vi "Message Logger.vi"() -> ()   [LabVIEW 2011, in "Messenging.lvlib" / "Message Logger.lvclass"]
uses:
  Message Logger.lvclass
  Parallel Process.lvclass
  Interprocess Messenger/Receiver/MGR (Receive type).lvclass
  Interprocess Messenger/TextVarientMessage/MSG.lvclass
  MessageLoggerMessage/MessageLoggerMessage.lvclass
  <vilib>/Utility/miscctls.llb/LVRowAndColumnUnsignedTypeDef.ctl
  Interprocess Messenger/Send/Send.lvclass
panel:
  out "Table":string[][](table)
  in  "Startup Message":refnum<class "MSG.lvclass">
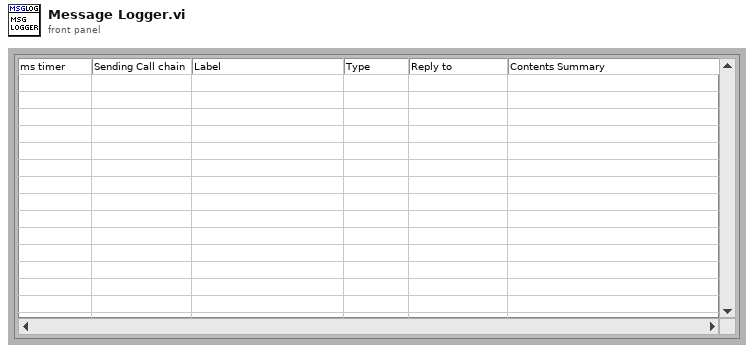
[diagram p1: front panel]
types:
  T1 = typedef "LVRowAndColumnUnsignedTypeDef.ctl" = cluster{"Row":u32, "Column":u32}
  T2 = cluster{"Timeout":i32, "Table":string[][], "index":i32}
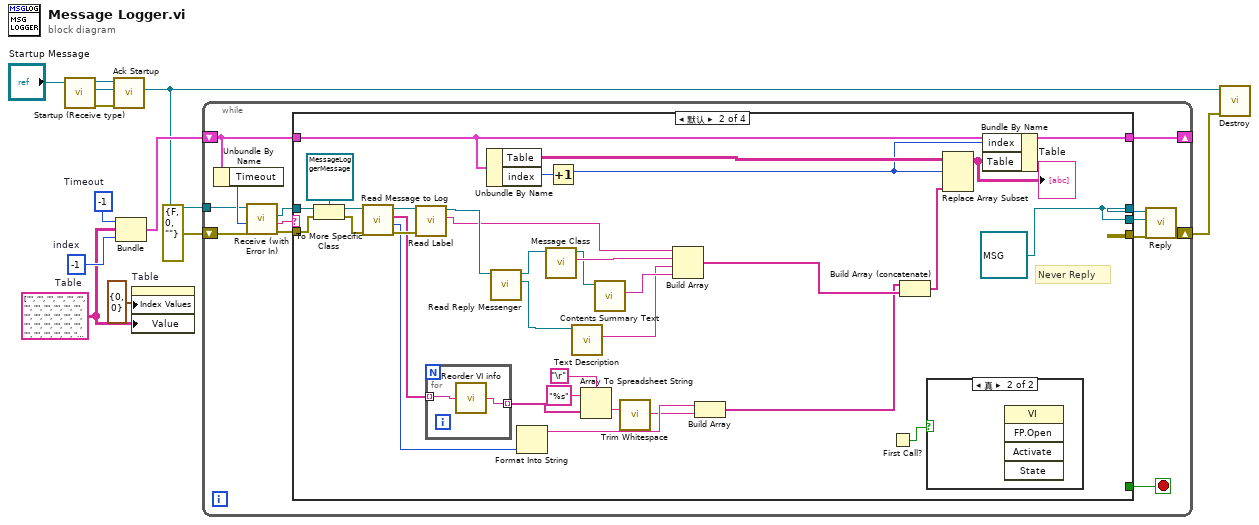
[diagram p0: block diagram]
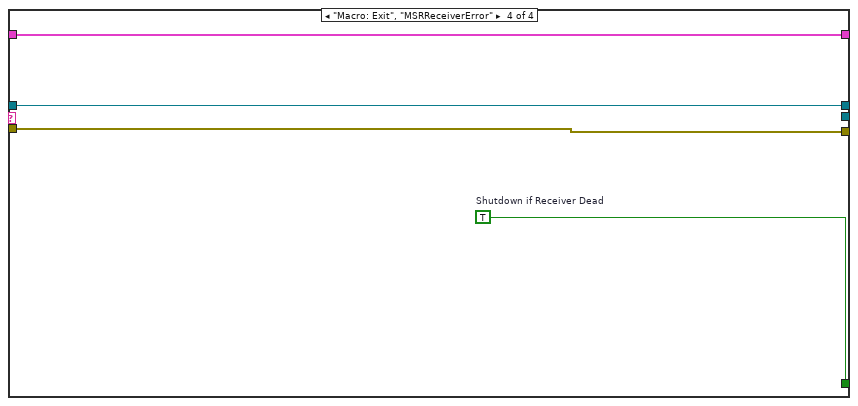
[diagram p5: hidden frame]
diagram:
  w3 = string[][] [["", "", "", "", "", ""], ["", "", "", "", "", ""], ["", "", "", "", "", ""], ["", "", "", "", "", ""], ["", "", "", "", "", ""], ["", "", "", "", "", ""], ["", "", "", "", "", ""], ["", "", "", "", "", ""], ["", "", "", "", "", ""], ["", "", "", "", "", ""], ["", "", "", "", "", ""], ["", "", "", "", "", ""], ["", "", "", "", "", ""], ["", "", "", "", "", ""], ["", "", "", "", "", ""], ["", "", "", "", "", ""], ["", "", "", "", "", ""], ["", "", "", "", "", ""], ["", "", "", "", "", ""], ["", "", "", "", "", ""], ["", "", "", "", "", ""], ["", "", "", "", "", ""], ["", "", "", "", "", ""], ["", "", "", "", "", ""], ["", "", "", "", "", ""], ["", "", "", "", "", ""], ["", "", "", "", "", ""], ["", "", "", "", "", ""], ["", "", "", "", "", ""], ["", "", "", "", "", ""], ["", "", "", "", "", ""], ["", "", "", "", "", ""], ["", "", "", "", "", ""], ["", "", "", "", "", ""], ["", "", "", "", "", ""], ["", "", "", "", "", ""], ["", "", "", "", "", ""], ["", "", "", "", "", ""], ["", "", "", "", "", ""], ["", "", "", "", "", ""], ["", "", "", "", "", ""], ["", "", "", "", "", ""], ["", "", "", "", "", ""], ["", "", "", "", "", ""], ["", "", "", "", "", ""], ["", "", "", "", "", ""], ["", "", "", "", "", ""], ["", "", "", "", "", ""], ["", "", "", "", "", ""], ["", "", "", "", "", ""], ["", "", "", "", "", ""], ["", "", "", "", "", ""], ["", "", "", "", "", ""], ["", "", "", "", "", ""], ["", "", "", "", "", ""], ["", "", "", "", "", ""], ["", "", "", "", "", ""], ["", "", "", "", "", ""], ["", "", "", "", "", ""], ["", "", "", "", "", ""], ["", "", "", "", "", ""], ["", "", "", "", "", ""], ["", "", "", "", "", ""], ["", "", "", "", "", ""], ["", "", "", "", "", ""], ["", "", "", "", "", ""], ["", "", "", "", "", ""], ["", "", "", "", "", ""], ["", "", "", "", "", ""], ["", "", "", "", "", ""], ["", "", "", "", "", ""], ["", "", "", "", "", ""], ["", "", "", "", "", ""], ["", "", "", "", "", ""], ["", "", "", "", "", ""], ["", "", "", "", "", ""], ["", "", "", "", "", ""], ["", "", "", "", "", ""], ["", "", "", "", "", ""], ["", "", "", "", "", ""], ["", "", "", "", "", ""], ["", "", "", "", "", ""], ["", "", "", "", "", ""], ["", "", "", "", "", ""], ["", "", "", "", "", ""], ["", "", "", "", "", ""], ["", "", "", "", "", ""], ["", "", "", "", "", ""], ["", "", "", "", "", ""], ["", "", "", "", "", ""], ["", "", "", "", "", ""], ["", "", "", "", "", ""], ["", "", "", "", "", ""], ["", "", "", "", "", ""], ["", "", "", "", "", ""], ["", "", "", "", "", ""], ["", "", "", "", "", ""], ["", "", "", "", "", ""], ["", "", "", "", "", ""], ["", "", "", "", "", " "]]  # Table
  w4 = -1  # index
  w9 = -1  # Timeout
  n1 = call "Startup (Receive type).vi"("Startup Message"="Startup Message") -> ("error out"=w6:errorcluster, "Command Messenger out"=w7:refnum<class "MGR (Receive type).lvclass">, "Starup Message"=w12:refnum<class "MSG.lvclass">)  [unwired: 1 in, 7 out]
  n2 = call "Ack Startup.vi"("error in"=w6, "Command Messenger"=w7, "Starup Message"=w12) -> ("Command Messenger"=w5:refnum<class "MGR (Receive type).lvclass">)  [unwired: 3 in, 5 out]
  n3 = Bundle("Timeout"=w9, "Table"=w3, "index"=w4) -> (w8:T2)  [unwired: 1 out]
  n4 = property on="Table" class="Tbl (严格)"("Index Values"=T1 {"Row"=0, "Column"=0}, "Value"=w3) -> ()  [unwired: 2 in, 2 out]
  n5 = while {
    shift-right: [w20] -> w10
    shift-left: errorcluster {"status"=FALSE, "code"=0, "source"=""} ("error out") -> [w22]
    shift-right: [w16] -> _
    shift-left: w8 -> [w15]
    tunnel: w5 -> [w14]
    stop <- w18 stop-if-true
    n6 = Unbundle By Name(w15) -> ("Timeout"=w17:i32)
    n7 = call-dynamic "Receive (with Error In).vi"("error in (no error)"=w22, "timeout in ms (5000)"=w17, "MGR in"=w14) -> ("error out"=w24:errorcluster, "Label"=w25:string, "Message"=w23:refnum<class "MSG.lvclass">)  [unwired: 6 out]
    n8 = case shown="默认" w25 {
      tunnel: w24 -> [w28 w50 w65 w68]
      tunnel: w23 -> [w27 w53 w67 w71]
      tunnel: [w28 _ w65 w68] -> w19
      tunnel: [w27 w55 w67 w71] -> w21
      tunnel: [_ _ _ w69] -> w18
      tunnel: [w26 w61 w66 w70] -> w16
      tunnel: w15 -> [w26 w62 w66 w70]
      tunnel: [_ w55 _ _] -> w13
      frame "------- Core ----------" {
        # "Core Cases for template"
      }
      frame Default {
        w55 = refnum<class "MSG.lvclass"> refnum ("Message")
        # "Never Reply"
        n9 = To More Specific Class(target class=refnum<class "MessageLoggerMessage.lvclass"> refnum ("Parallel Process.lvlib:MessageLoggerMessage.lvclass"), reference=w53, error in=w50) -> (specific class reference=w49:refnum<class "MessageLoggerMessage.lvclass">, error out=w48:errorcluster)
        n10 = call "Read Message to Log.vi"("error in (no error)"=w48, "MessageLoggerMessage.lvclass in"=w49) -> ("error out"=w47:errorcluster, "millisecond timer"=w44:u32, "call chain"=w37:string[], "Messenging.lvlib:Interprocess Message"=w46:refnum<class "MSG.lvclass">)  [unwired: 6 out]
        n11 = call-dynamic "Read Label.vi"("error in (no error)"=w47, "Message"=w46) -> ("Label"=w51:string, "Message"=w52:refnum<class "MSG.lvclass">)  [unwired: 8 out]
        n12 = for {
          tunnel: w37 -> [w64] mode=indexing
          tunnel: [w63] -> w36 mode=indexing
          n13 = call "Reorder VI info.vi"("chain"=w64) -> ("Reorderded"=w63:string)
        }
        n14 = Unbundle By Name(w62) -> ("Table"=w60:string[][], "index"=w59:i32)
        n15 = call-dynamic "Read Reply Messenger.vi"("Messege"=w52) -> ("Reply to..."=w31:refnum<class "Send.lvclass">, "Message"=w32:refnum<class "MSG.lvclass">)  [unwired: 1 in, 8 out]
        n16 = Format Into String(w44) -> (resulting string=w43:string)  [unwired: 3 in, 1 out]
        n17 = call-dynamic "Message Class.vi"("Message"=w32) -> ("Message Class"=w35:string, "Message"=w34:refnum<class "MSG.lvclass">)  [unwired: 1 in, 8 out]
        n18 = Increment(x=w59) -> (x+1=w58:i32)
        n19 = call-dynamic "Text Description.vi"("Send in"=w31) -> ("Description"=w30:string)  [unwired: 10 out]
        n20 = Array To Spreadsheet String(delimiter (Tab)="\r", array=w36, 3:"%s" ("format string")) -> (spreadsheet string=w42:string)
        n21 = call-dynamic "Contents Summary Text.vi"("Message"=w34) -> ("Contents Summary Text"=w33:string)  [unwired: 10 out]
        n22 = call <vilib>:"Trim Whitespace.vi"("string"=w42) -> ("trimmed string"=w38:string)  [unwired: 1 in]
        n23 = Build Array(w51, w35, w30, w33) -> (w57:string[])
        n24 = Build Array(w43, w38) -> (w39:string[])
        n25 = First Call?() -> (First Call?: T/F=w29:bool)
        n26 = Build Array (concatenate)(w39, w57) -> (w41:string[])
        n27 = case shown="真" w29 {
          frame False {
          }
          frame True {
            n28 = invoke class="VI" method="FP.Open"() -> ()  [unwired: 5 in, 5 out]
          }
        }
        n29 = Replace Array Subset(array=w60, new element=w41, index (row)=w58) -> (w56:string[][])  [unwired: 1 in]
        "Table" <- w56
        n30 = Bundle By Name(cluster=w62, "index"=w58, "Table"=w56) -> (w61:T2)
      }
      frame "MSRReceiveTimedOut" {
      }
      frame "Macro: Exit", "MSRReceiverError" {
        w69 = TRUE  # Shutdown if Receiver Dead
      }
    }
    n31 = call-dynamic "Reply.vi"("error in (no error)"=w19, "Reply"=w13, "Message to Reply to"=w21) -> ("error out"=w20:errorcluster)  [unwired: 8 out]
  }
  n32 = call-dynamic "Destroy.vi"("error in (no error)"=w10, "Messenger in"=w5) -> ()  [unwired: 10 out]
